vi "Job reference.vi"(8 "error in (no error)":errorcluster, 11 "VGS_Job in":refnum<class "VGS_Job.lvclass">) -> (0 "error out":errorcluster, 2 "Job reference":refnum<k24>, 3 "VGS_Job out":refnum<class "VGS_Job.lvclass">)   [LabVIEW 2022 SP3, in "LV_VGS.lvlib" / "VGS_Job.lvclass"]
uses:
  VGS_Job.lvclass
  C:/Users/Andrey/Documents/GitHub/LV_VGS/vgs_project.dll
  vgs_project.dll
  VGS_Job.lvclass/VGS_Job.ctl
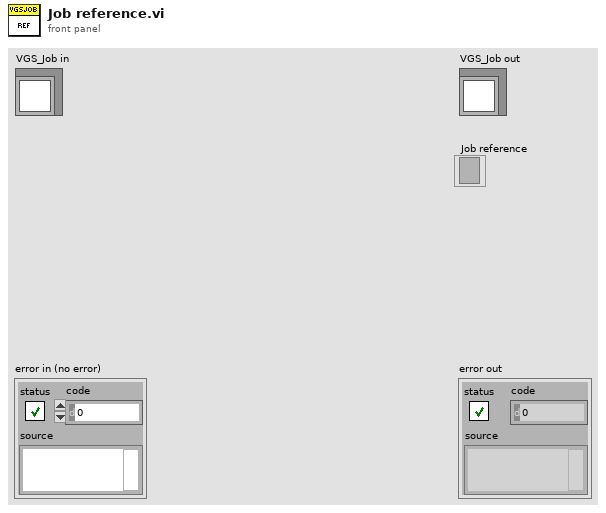
[diagram p1: front panel]
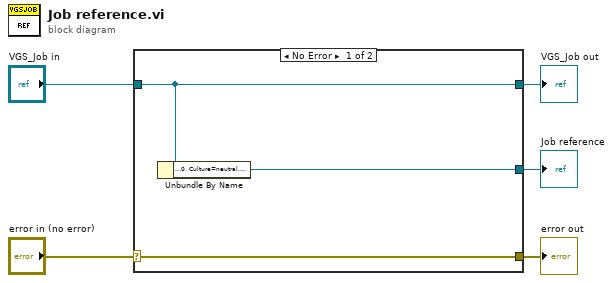
[diagram p0: block diagram]
diagram:
  n1 = case shown="No Error" "error in (no error)" {
    selector: "error in (no error)" -> [w8 w9]
    tunnel: [w8 w9] -> w4
    tunnel: [w7 w10] -> w2
    tunnel: "VGS_Job in" -> [w7 w10]
    tunnel: [w6 _] -> w1
    frame No Error {
      n2 = Unbundle By Name(w7) -> ("Job reference"=w6:refnum<k24>)
    }
    frame Error {
    }
  }
  "error out" <- w4
  "VGS_Job out" <- w2
  "Job reference" <- w1
